vi "Octal Channel Test Panel.vi"() -> ()   [LabVIEW 2016]
uses:
  Program Files/Crystal Technology/Developer/AotfLibrary/Dll/AotfLibrary.dll
panel:
  in  "Clear Display":bool
  out "Connected":bool
  in  "AOTF Index":i32
  in  "Quit":bool
  in  "Send Command":bool
  out "AOTF Response":string
  in  "AOTF Command":string
  # "Example Commands\n\nGet device info\nBoardID\n\nSet frequency for channel 0\ndds f 0 86.130500\n\nSet power level for channel 0 (max is 16383)\ndds a 0 16300\n\nTurn off channel 0\ndds a 0 0"
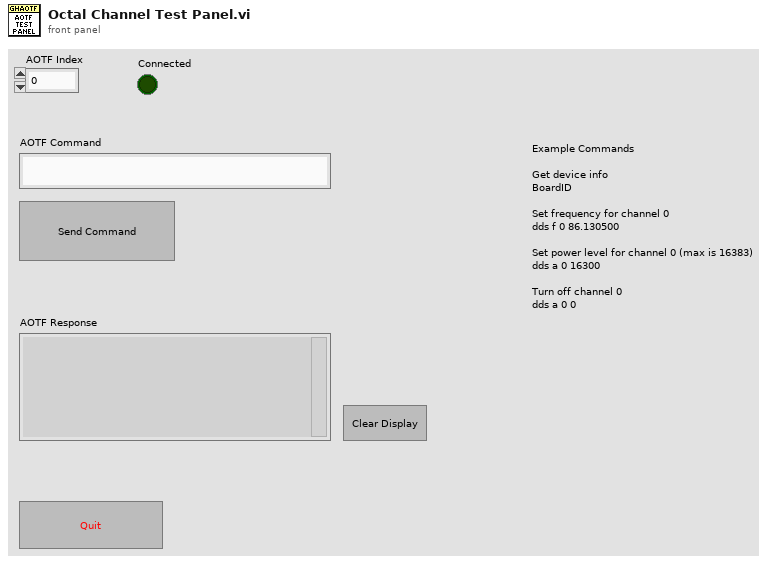
[diagram p1: front panel]
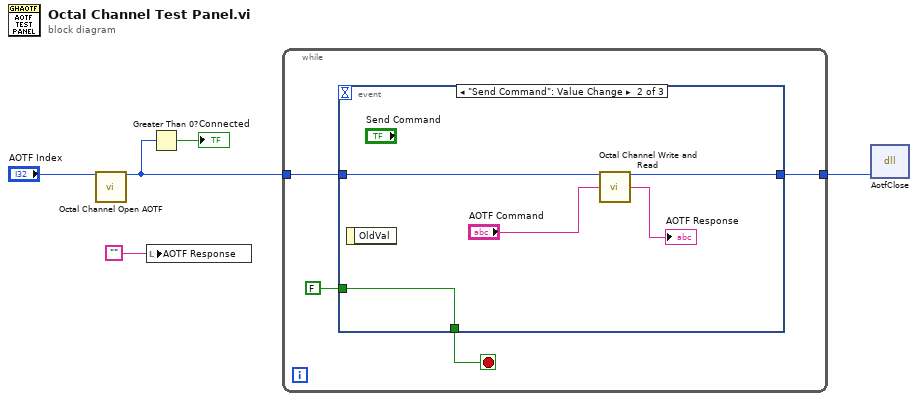
[diagram p0: block diagram]
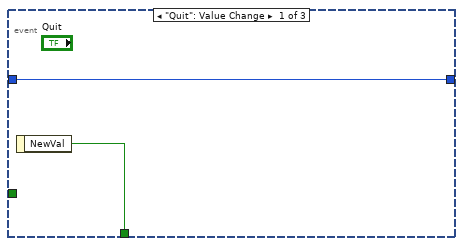
[diagram p2: hidden frame]
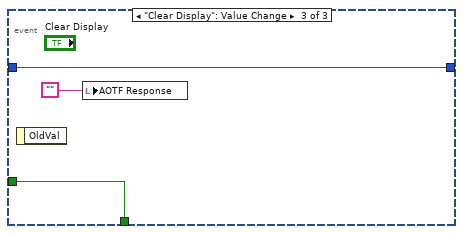
[diagram p3: hidden frame]
diagram:
  n1 = call "Octal Channel Open AOTF.vi"("AOTF Index"="AOTF Index") -> ("AOTF Handle"=w3:u64)  [unwired: 13 in, 1 out]
  n2 = local write "AOTF Response"("") -> ()
  n3 = Greater Than 0?(x=w3) -> (x > 0?=→"Connected":bool)
  n4 = while {
    tunnel: w3 -> [w7]
    tunnel: [w6] -> w4
    stop <- w9 stop-if-true
    n5 = event shown="[1] \"Send Command\": Value Change" {
      selector: _ -> [_ _ _]
      dyn-events: _ -> [_ _ _]
      timeout: _ -> [_ _ _]
      tunnel: [w11 w16 w19] -> w9
      tunnel: FALSE -> [_ w16 w19]
      tunnel: w7 -> [w10 w15 w17]
      tunnel: [w10 w12 w17] -> w6
      event "Quit": Value Change {
        n6 = event-data() -> ("NewVal"=w11:bool)  [unwired: 1 in]
      }
      event "Send Command": Value Change {
        n7 = event-data() -> ()  [unwired: 1 in, 1 out]
        n8 = call "Octal Channel Write and Read.vi"("hAotfController"=w15, "Command"="AOTF Command") -> ("hAotfController (Dup)"=w12:u64, "Response"=→"AOTF Response":string)  [unwired: 11 in, 1 out]
      }
      event "Clear Display": Value Change {
        n9 = event-data() -> ()  [unwired: 1 in, 1 out]
        n10 = local write "AOTF Response"("") -> ()
      }
    }
  }
  n11 = dll-call lib="C:/Program Files/Crystal Technology/Developer/AotfLibrary/Dll/AotfLibrary.dll" fn="AotfClose"("hAotfContoller"=w4) -> ()  [unwired: 5 in, 2 out]
